vi "Select Serial Port.vi"() -> (3 "VISA资源名称 2":refnum<visa-resource-name>)   [LabVIEW 2015, in "Debug.lvlib"]
uses:
  Debug.lvlib
panel:
  in  "确定按钮":bool
  in  "VISA资源名称":refnum<visa-resource-name>
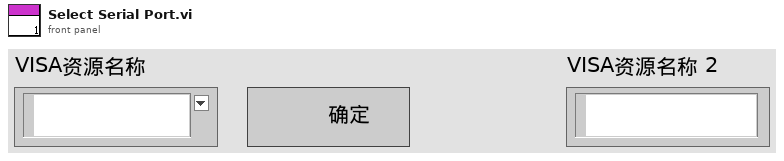
[diagram p1: front panel]
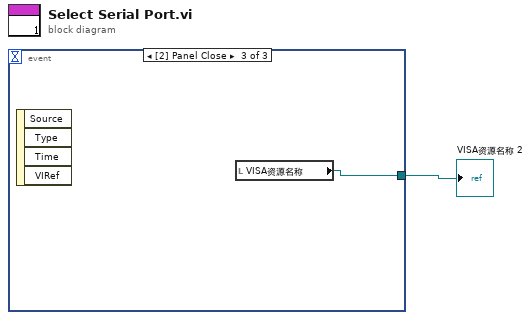
[diagram p0: block diagram]
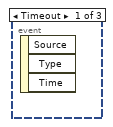
[diagram p2: hidden frame]
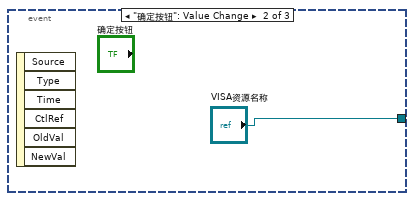
[diagram p3: hidden frame]
diagram:
  n1 = event shown="[2] Panel Close" {
    selector: _ -> [_ _ _]
    dyn-events: _ -> [_ _ _]
    timeout: _ -> [_ _ _]
    tunnel: [_ "VISA资源名称" w3] -> w1
    event Timeout {
      n2 = event-data() -> ()  [unwired: 1 in, 3 out]
    }
    event "确定按钮": Value Change {
      n3 = event-data() -> ()  [unwired: 1 in, 6 out]
    }
    event Panel Close {
      n4 = event-data() -> ()  [unwired: 1 in, 4 out]
      n5 = local read "VISA资源名称"() -> (w3:refnum<visa-resource-name>)
    }
  }
  "VISA资源名称 2" <- w1
